vi "Dashboard Main.vi"() -> ()   [LabVIEW 2015]
uses:
  <vilib>/Utility/miscctls.llb/LVRowAndColumnTypeDef.ctl
  <vilib>/event_ctls.llb/eventvkey.ctl
  <vilib>/Rock Robotics/WPI/Dashboard/WPI_DashboardLogging Global.vi
  <vilib>/Utility/config.llb/Write Key (String).vi
  <vilib>/Utility/config.llb/Write Key (I32).vi
  <vilib>/Utility/config.llb/NI_LVConfig.lvlib
panel:
  in  "TCP":refnum<k5>
  in  "Rec Mode":enum32{"Stop", "Record", "Playback"}(radio)
  in  "Vision":u16(ring)=2 items=["Camera Off", "USB Camera SW", "USB Camera HW", "IP Camera"]
  out "Camera IP":string
  out "Image Message":string="Timeout in Camera Communications"
  in  "Dashboard Tab":T1(tab)
  out "Ball in Intake Arm":bool
  in  "Vertical Line (Pixels)":dbl=179.0
  in  "Horizonal Line (Pixels)":dbl=164.0
  in  "Select Auto":string(combo)
  out "NT Connection":bool
  in  "Camera Settings":T2={"Frame Rate"=30, "Compression"=30, "Size"=1} {"Frame Rate" scale=1.0..30.0; "Size" items=["640x480", "320x240", "160x120"]}
  out "Mode":T3(ring)=enum."Auto Disabled"
  in  "DB Camera Config":bool
  out "fps":dbl format="%#.1g"
  out "Mbps":dbl format="%#.1g"
  out "Mbps LED":bool
  in  "Crosshair Color":u32(colorbox)=782080
  out "net address":u32
  out "Numeric":i32
  in  "DB/String 9":string
  in  "DB/String 8":string
  in  "DB/String 7":string
  in  "DB/String 6":string
  in  "DB/String 5":string
  in  "DB/String 4":string
  in  "DB/String 3":string
  in  "DB/String 2":string
  in  "DB/String 1":string
  in  "DB/String 0":string
  in  "DB/Slider 0":dbl(slide) scale=0.0..5.0
  in  "DB/Slider 1":dbl(slide) scale=0.0..5.0
  in  "DB/Slider 2":dbl(slide) scale=0.0..5.0
  in  "DB/Slider 3":dbl(slide) scale=0.0..5.0
  out "DB/LED 3":bool
  out "DB/LED 2":bool
  out "DB/LED 1":bool
  out "DB/LED 0":bool
  in  "DB/Button 3":bool
  in  "DB/Button 2":bool
  in  "DB/Button 1":bool
  in  "DB/Button 0":bool caption="New Name"
  in  "Test Slider":dbl(slide) scale=0.0..100.0 scale format="%#_3g"
  in  "On/Off":bool caption="Solenoid"
  in  "Test Name":u16(ring) items=["Select the test to run..."]
  in  "Test Tree":string(tree)
  in  "Motor":cluster{"Value":dbl, "Enable":bool} {"Value" scale=-1.0..1.0 scale format="%#_3g"}
  out "Progress":T4 {"Test Progress" scale=0.0..100.0}
  in  "Rev/Fwd":cluster{"Forward":bool, "Reverse":bool}
  in  "Test Ring":u16(ring) items=["Monochrome", "Color"]
  out "Cmd Status":string
  in  "Execute Command":bool
  in  "Command Params":string[][](table)
  in  "Command Selection":i32(listbox)
  in  "CheckList":i32(listbox)
  out "Tree":string(tree)
  out "Camera Image":T5(plugin-control)
  out "Background":bool
  # "This tab is a great place for autonomous settings and robot-specific values.\nPlace controls and indicators inside this tab and match name to\nDashboard Variables on robot. You can also delete this comment."
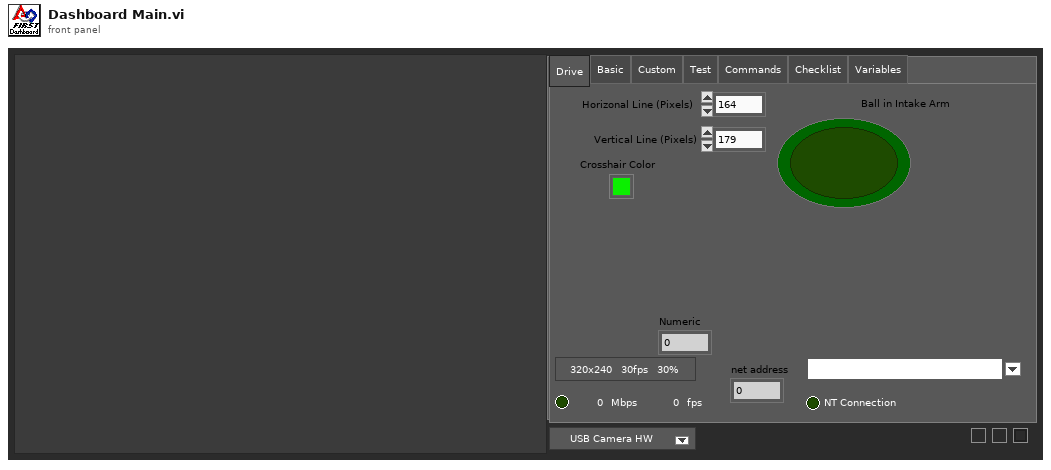
[diagram p1: front panel]
types:
  T1 = enum32{"Drive", "Basic", "Custom", "Test", "Commands", "Checklist", "Variables"}
  T2 = cluster{"Frame Rate":i32, "Compression":i32, "Size":u16}
  T3 = enum8{"Tele-Op Disabled", "Tele-Op Enabled", "Auto Disabled", "Auto Enabled", "Test Disabled", "Test Enabled", "Disconnected", "No Code", "E-Stop"}
  T4 = cluster{"Test Progress":u8, "Test Progress Text":string}
  T5 = typedef "IMAQ Image.ctl" = refnum<image>
  T6 = cluster{"IDs":cluster{"RPC field ID":u16, "Unique ID":u16}, "String":string}
  T7 = enum32{"Drive", "Basic", "Custom", "Test", "Checklist", "Variables"}
  T8 = typedef "Image Type" = u32
  T9 = cluster{"Camera Image":refnum<vi>, "Dashboard Tab":refnum<vi>, "Background":refnum<vi>, "Vision":refnum<vi>, "Rec Mode":refnum<vi>, "Test Slider":refnum<vi>, "On/Off ":refnum<vi>, "Test Ring":refnum<vi>, "Rev/Fwd":refnum<vi>, "Test Name":refnum<vi>, "Motor":refnum<vi>, "Progress":refnum<vi>, "CheckList":refnum<vi>, "Tree":refnum<vi>, "Test Tree":refnum<vi>, "Command Params":refnum<vi>, "Command Selection":refnum<vi>, "Execute Command":refnum<vi>, "Cmd Status":refnum<vi>}
  T10 = cluster{"Error Strings":string, "Disable Counts":cluster{u16, u16}, "Rail Faults":cluster{u16, u16, u16}, "Robot IP":string, "DB Mode":u8, "Event Info":cluster{"Name":string, "Type":u8, "Number":u16, "Replay":u8}, "Camera Addr":string}
  T11 = cluster{"Storage":cluster{"Disk Free":u64, "RAM Block":u32, "RAM free":u32}, "CPU Utilization":cluster{"CPU % ISR":sgl, "CPU % Time Crit":sgl, "CPU % Timed Str":sgl, "CPU % High":sgl, "CPU % Above":sgl, "CPU % Normal":sgl, "CPU % Low":sgl}, "CAN":cluster{"% Bus Utilization":sgl, "Bus Off Cnt":u32, "TX_FIFO Full Cnt":u32, "Receive Error Cnt":u8, "Transmit Error Cnt":u8}, "HID":cluster{"HID Outputs":u32, "Rumble Low":u16, "Rumble High":u16}[]}
  T12 = cluster{"Status bits":cluster{"Test Mode":bool, "Autonomous":bool, "Enabled":bool, "Code Start":bool, "Brownout":bool, "Reserved 2":bool, "Reserved 3":bool, "E-Stop":bool}, "Code Trace":cluster{"Disabled":bool, "TeleOp":bool, "Auto":bool, "Test":bool}, "Controller Type":enum16{"unknown", "cRIO", "roboRio"}, "Code?":enum16{"unknown", "noCode", "code"}, "Battery V":dbl}
  T13 = cluster{"Control Bits":cluster{"TestMode":bool, "Autonomous":bool, "Enabled":bool, "FMS Present":bool, bool, bool, bool, "E-Stop":bool}, "Team Station ":u8, "Countdown":sgl, "Joystick Values":cluster{"Axes":dbl[], "Buttons":bool[], "POVs":i16[]}[]}
  T14 = cluster{"Horizonal Line (Pixels)":dbl, "Horizonal Line (Pixels)":dbl}
  T15 = cluster{"Horizonal Line (Pixels)":dbl, "Vertical Line (Pixels)":dbl}
  T16 = typedef "NI_LVConfig.lvlib/Config Data RefNum.ctl" = refnum<k1>
  T17 = cluster{"Operation":enum16{"Update", "Clear"}, "Color Box":u32}[]
  T18 = typedef "eventvkey.ctl" = enum16{"ASCII", "Enter", "Return", "Shift", "Ctrl", "Alt", "Cmd", "Opt", "Caps", "NumLock", "Clear", "Break", "Up", "Down", "Left", "Right", "Insert", "Delete", "Home", "End", "PageUp", "PageDown", "Escape", "Help", "Pause", "ScrollLock", "F1", "F2", "F3", "F4", "F5", "F6", "F7", "F8", "F9", "F10", "F11", "F12", "F13", "F14", "F15", "F16", "F17", "F18", "F19", "F20", "F21", "F22", "F23", "F24", "Play", "VolumeUp", "VolumeDown", "Mute", "Two Byte Char"}
  T19 = cluster{"Image Size":bool, "Image Type":bool, "Pixel Value":bool, "ROI Information":bool, "Zoom Factor":bool}
  T20 = enum8{"Enabled", "Disabled", "Disabled and Grayed Out"}
  T21 = cluster{"Operation":enum16{"Update", "Clear"}, "Color Box":u32}
  T22 = typedef "LVRowAndColumnTypeDef.ctl" = cluster{"Row":i32, "Column":i32}
  T23 = cluster{"Shift":bool, "Ctrl":bool, "Alt":bool, "Cmd":bool, "Opt":bool}
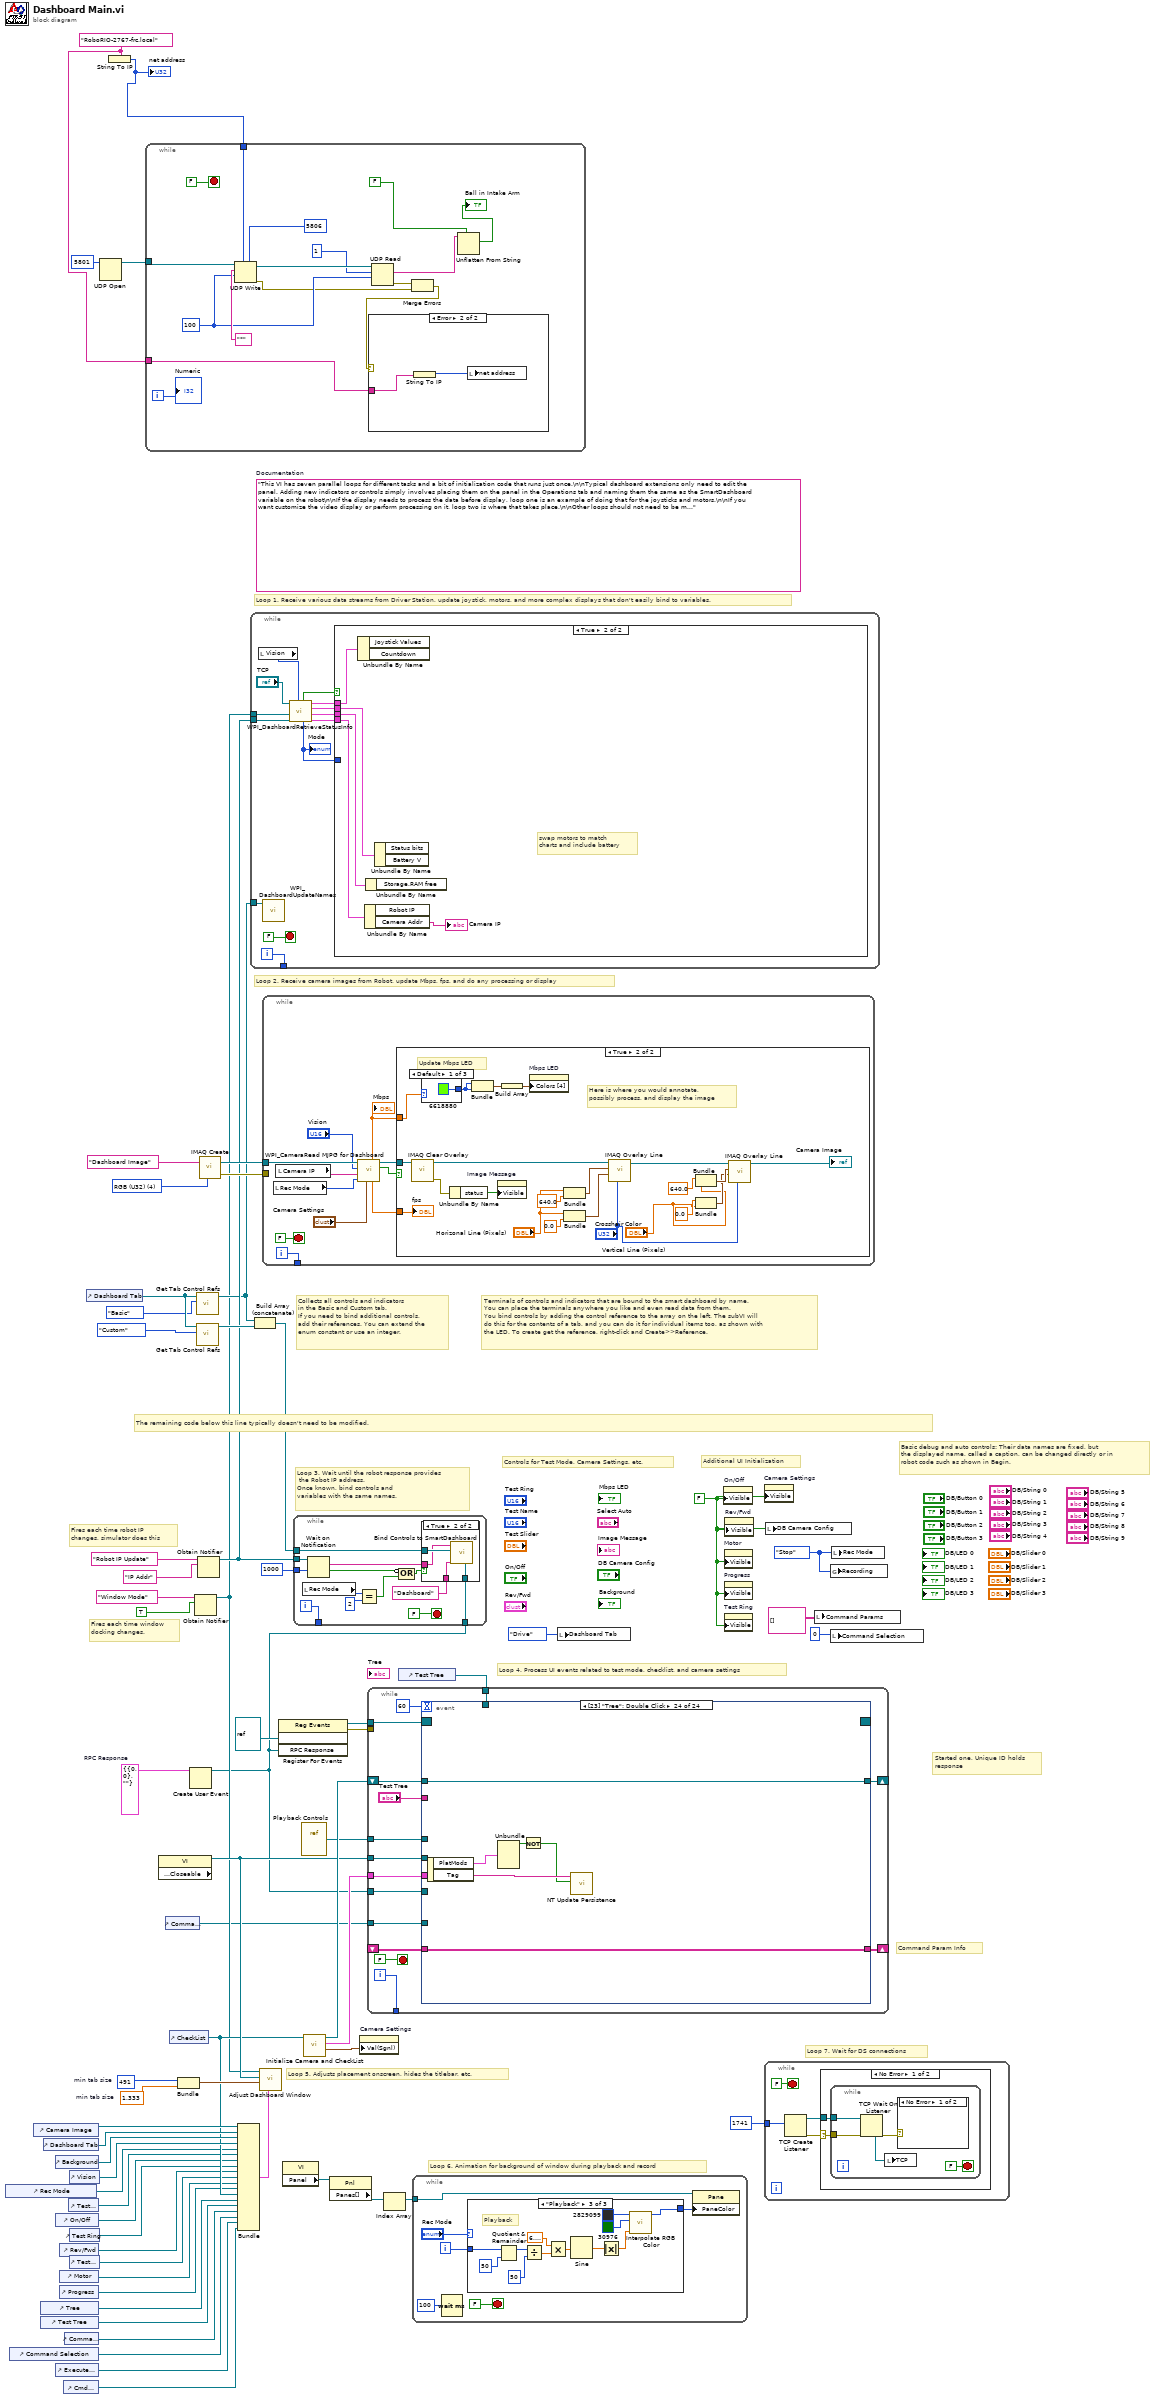
[diagram p0: block diagram]
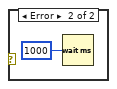
[diagram p3: hidden frame]
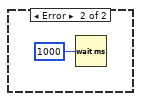
[diagram p4: hidden frame]
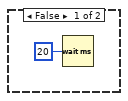
[diagram p5: hidden frame]
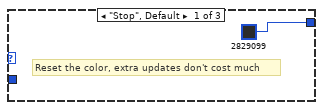
[diagram p6: hidden frame]
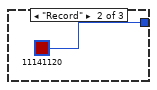
[diagram p7: hidden frame]
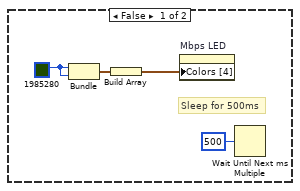
[diagram p9: hidden frame]
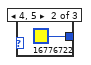
[diagram p10: hidden frame]
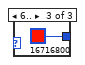
[diagram p11: hidden frame]
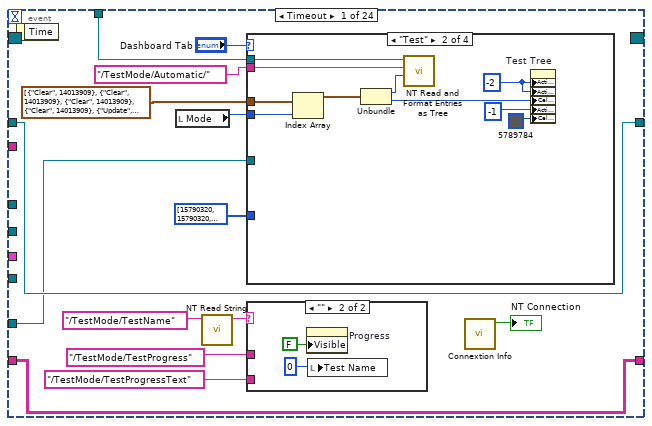
[diagram p12: hidden frame]
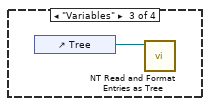
[diagram p14: hidden frame]
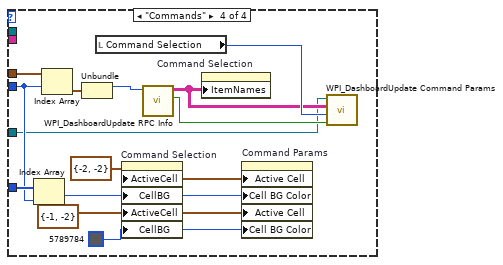
[diagram p15: hidden frame]
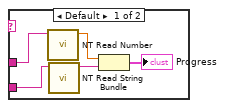
[diagram p16: hidden frame]
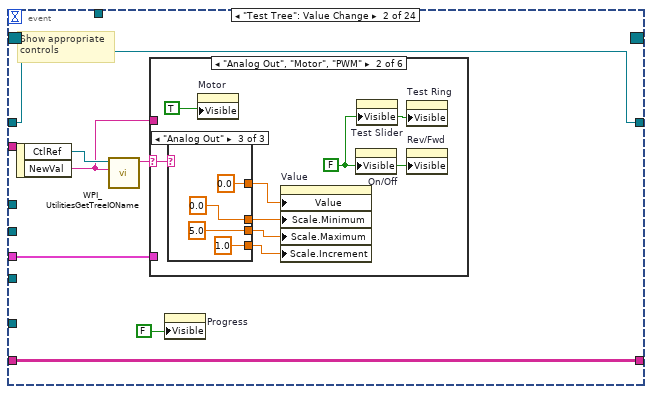
[diagram p17: hidden frame]
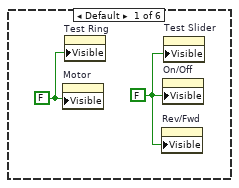
[diagram p18: hidden frame]
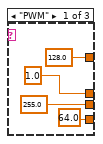
[diagram p19: hidden frame]
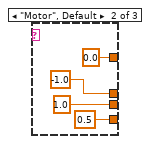
[diagram p20: hidden frame]
diagram:
  w1 = "RoboRIO-2767-frc.local" ("name")
  w11 = T6 {"IDs"={"RPC field ID"=0, "Unique ID"=0}, "String"=""}  # RPC Response
  w37 = 491  # min tab size
  w36 = 1.333  # min tab size
  w45 = enum32{"Stop", "Record", "Playback"}."Stop" ("Rec Mode")
  w19 = FALSE ("Visible")
  (unwired) "This VI has seven parallel loops for different tasks and a bit of initialization code that runs just once.\n\nTypical dashboard extensions only need to edit the panel. Adding new indicators or controls simply involves placing them on the panel in the Operations tab and naming them the same as the SmartDashboard variable on the robot\n\nIf the display needs to process the data before display, loop one is an example of doing that for the joysticks and motors.\n\nIf you want customize the video display or perform processing on it, loop two is where that takes place.\n\nOther loops should not need to be modified. They are pretty standard, and document the task they perform."  # Documentation
  w65 = T8 4 items=["Grayscale (U8)", "Grayscale (I16)", "Grayscale (SGL)", "Complex (CSG)", "RGB (U32)", "HSL (U32)", "RGB (U64)"] ("Image Type")
  # "Command Param Info"
  # "Started one, Unique ID holds\nresponse"
  # "Loop 7. Wait for DS connections"
  # "Basic debug and auto controls: Their data names are fixed, but\nthe displayed name, called a caption, can be changed directly or in\nrobot code such as shown in Begin."
  # "Controls for Test Mode, Camera Settings, etc."
  # "Additional UI Initialization"
  # "Loop 6. Animation for background of window during playback and record"
  # "Fires each time robot IP\nchanges, simulator does this"
  # "Fires each time window\ndocking changes."
  # "Collects all controls and indicators\nin the Basic and Custom tab.\nIf you need to bind additional controls,\nadd their references. You can extend the\nenum constant or use an integer."
  # "The remaining code below this line typically doesn't need to be modified."
  # "Loop 4. Process UI events related to test mode, checklist, and camera settings"
  # "Terminals of controls and indicators that are bound to the smart dashboard by name.\nYou can place the terminals anywhere you like and even read data from them.\nYou bind controls by adding the control reference to the array on the left. The subVI will\ndo this for the contents of a tab, and you can do it for individual items too, as shown with\nthe LED. To create get the reference, right-click and Create>>Reference."
  # "Loop 3. Wait until the robot response provides\n the Robot IP address.\nOnce known, bind controls and\nvariables with the same names."
  # "Loop 5. Adjusts placement onscreen, hides the titlebar, etc."
  # "Loop 1. Receive various data streams from Driver Station, update joystick, motors, and more complex displays that don't easily bind to variables."
  # "Loop 2. Receive camera images from Robot, update Mbps, fps, and do any processing or display"
  n1 = control-ref of="Rec Mode"() -> (w25:refnum<vi>)
  n2 = control-ref of="Command Selection"() -> (w10:refnum<vi>)
  n3 = control-ref of="Camera Image"() -> (w40:refnum<vi>)
  n4 = control-ref of="Tree"() -> (w29:refnum<vi>)
  n5 = control-ref of="Test Tree"() -> (w28:refnum<vi>)
  n6 = control-ref of="Dashboard Tab"() -> (w39:refnum<vi>)
  n7 = control-ref of="Execute Command"() -> (w12:refnum<vi>)
  n8 = control-ref of="Background"() -> (w34:refnum<vi>)
  n9 = control-ref of="On/Off"() -> (w23:refnum<vi>)
  n10 = control-ref of="Progress"() -> (w20:refnum<vi>)
  n11 = control-ref of="Rev/Fwd"() -> (w21:refnum<vi>)
  n12 = control-ref of="Motor"() -> (w26:refnum<vi>)
  n13 = control-ref of="Cmd Status"() -> (w6:refnum<vi>)
  n14 = control-ref of="Command Params"() -> (w13:refnum<vi>)
  n15 = control-ref of="Test Slider"() -> (w24:refnum<vi>)
  n16 = control-ref of="Vision"() -> (w38:refnum<vi>)
  n17 = control-ref of="Test Ring"() -> (w22:refnum<vi>)
  n18 = control-ref of="Test Name"() -> (w27:refnum<vi>)
  n19 = control-ref of="Dashboard Tab"() -> (w43:refnum<vi>)
  n20 = UDP Open(11:u16 5801 ("port")) -> (port=w3:refnum<k16>)  [unwired: 4 in, 2 out]
  n21 = String To IP(1:w1) -> (0:w2:u32)
  "net address" <- w2
  n22 = while {
    tunnel: w3 -> [w79]
    tunnel: w2 -> [w70]
    tunnel: w1 -> [w66]
    i -> [w72]
    stop <- FALSE stop-if-true
    w71 = 100 ("timeout ms (25000)")
    n23 = UDP Write(address=w70, port or service name=u16 5806, connection ID=w79, data in="*", 9:w71) -> (error out=w68:errorcluster, 3:w77:refnum<k16>)  [unwired: 1 in]
    n24 = UDP Read(connection ID=w77, max size (548)=1, timeout ms (25000)=w71) -> (data out=w74:string, error out=w69:errorcluster)  [unwired: 1 in, 3 out]
    n25 = Merge Errors(w69, w68) -> (w67:errorcluster)
    n26 = case shown="Error" w67 {
      tunnel: w66 -> [_ w82]
      frame No Error {
      }
      frame Error {
        n27 = String To IP(1:w82) -> (0:w83:u32)
        n28 = local write "net address"(w83) -> ()
      }
    }
    n29 = Unflatten From String(type=FALSE ("Boolean"), binary string=w74) -> (value=→"Ball in Intake Arm":bool)  [unwired: 3 in, 2 out]
    "Numeric" <- w72
  }
  n30 = property class="VI" props=["Front Panel.Closeable"]() -> (reference out=w44:refnum<vi>)  [unwired: 2 in, 2 out]
  n31 = control-ref of="Command Params"() -> (w5:refnum<vi>)
  n32 = control-ref of="CheckList"() -> (w30:refnum<vi>)
  n33 = Bundle("min tab size"=w37, "min tab size"=w36) -> (w35:cluster{"min tab size":i32, "min tab size":dbl})  [unwired: 1 in]
  n34 = Create User Event(user event datatype=w11) -> (user event=w7:refnum<user-event>)  [unwired: 1 in, 1 out]
  n35 = Obtain Notifier(name (unnamed)="Window Mode", notification data type=TRUE) -> (notifier out=w16:refnum<notifier>)  [unwired: 2 in, 2 out]
  n36 = call <vilib>:"Get Tab Control Refs.vi"("Page Index"=T7."Basic" ("Dashboard Tab"), "TabControl in"=w43) -> ("ControlsOnPage"=w17:refnum<vi>[])  [unwired: 9 in]
  n37 = call <vilib>:"Get Tab Control Refs.vi"("Page Index"=T7."Custom" ("Dashboard Tab"), "TabControl in"=w43) -> ("ControlsOnPage"=w42:refnum<vi>[])  [unwired: 9 in]
  n38 = Obtain Notifier(name (unnamed)="Robot IP Update", notification data type="IP Addr" ("name (unnamed)")) -> (notifier out=w18:refnum<notifier>)  [unwired: 2 in, 2 out]
  n39 = call "IMAQ Create"("Image Name"="Dashboard Image", "Image Type"=w65) -> ("New Image"=w63:T5, "error out"=w62:errorcluster)  [unwired: 2 in, 1 out]
  n40 = Bundle("Camera Image"=w40, "Dashboard Tab"=w39, "Background"=w34, "Vision"=w38, "Rec Mode"=w25, "Test Slider"=w24, "On/Off"=w23, "Test Ring"=w22, "Rev/Fwd"=w21, "Test Name"=w27, "Motor"=w26, "Progress"=w20, "CheckList"=w30, "Tree"=w29, "Test Tree"=w28, "Command Params"=w13, "Command Selection"=w10, "Execute Command"=w12, "Cmd Status"=w6) -> (w31:T9)  [unwired: 1 in]
  n41 = while {
    tunnel: [w95] -> _
    tunnel: w18 -> [w89]
    tunnel: w17 -> [w88]
    tunnel: w16 -> [w84]
    i -> [w95]
    stop <- FALSE stop-if-true
    n42 = local read "Vision"() -> (w86:u16)
    n43 = call <vilib>:"WPI_DashboardUpdateNames.vi"("Controls on Tab"=w88) -> ()  [unwired: 11 in]
    n44 = call <vilib>:"WPI_DashboardRetrieveStatusInfo.vi"("Vision"=w86, "Binding Refnum"=w89, "Window Mode Notifier"=w84, "TCP Cnx"="TCP") -> ("Power and Errors"=w90:T10, "Robot Metrics"=w93:T11, "Status Info"=w94:T12, "Control Info"=w91:T13, "Robot Mode"=w87:T3, "Process?"=w92:bool)  [unwired: 2 in]
    "Mode" <- w87
    n45 = case shown="True" w92 {
      tunnel: w94 -> [_ w102]
      tunnel: w93 -> [_ w101]
      tunnel: w91 -> [_ w100]
      tunnel: w90 -> [_ w99]
      tunnel: w87 -> [_ _]
      frame False {
        n46 = Wait (ms)(milliseconds to wait=u32 20) -> ()  [unwired: 1 out]
      }
      frame True {
        # "swap motors to match\ncharts and include battery"
        n47 = Unbundle By Name(w100) -> ()  [unwired: 2 out]
        n48 = Unbundle By Name(w99) -> ("Camera Addr"=→"Camera IP":string)  [unwired: 1 out]
        n49 = Unbundle By Name(w101) -> ()  [unwired: 1 out]
        n50 = Unbundle By Name(w102) -> ()  [unwired: 2 out]
      }
    }
  }
  n51 = Build Array (concatenate)(w17, w42) -> (w41:refnum<vi>[])
  n52 = call "Adjust Dashboard Window.vi"("Sizing Refnums"=w31, "Size Constraints"=w35, "VI"=w44, "WIn Mode"=w16) -> ()  [unwired: 8 in]
  n53 = while {
    tunnel: w63 -> [w111]
    tunnel: w62 -> [_]
    tunnel: [w112] -> _
    i -> [w112]
    stop <- FALSE stop-if-true
    n54 = local read "Rec Mode"() -> (w106:enum32{"Stop", "Record", "Playback"})
    n55 = local read "Camera IP"() -> (w104:string)
    n56 = call <vilib>:"WPI_CameraRead MJPG for Dashboard.vi"("Camera Settings"="Camera Settings", "Rec Mode"=w106, "Camera IP"=w104, "Camera Mode"="Vision", "Refnum in"=w111) -> ("Active"=w109:bool, "Refnum out"=w110:T5, "FPS"=w108:dbl, "Bandwidth (Mbps)"=w103:dbl)  [unwired: 3 in]
    "Mbps" <- w103
    n57 = case shown="True" w109 {
      tunnel: w110 -> [_ w134]
      tunnel: w103 -> [_ w133]
      tunnel: w108 -> [_ w132]
      frame False {
        w114 = u32 1985280 ("Color Box")
        # "Sleep for 500ms"
        n58 = Bundle("Color Box"=w114, "Color Box"=w114) -> (w116:cluster{"Color Box":u32, "Color Box":u32})  [unwired: 1 out]
        n59 = Build Array(w116) -> (w115:cluster{"Color Box":u32, "Color Box":u32}[])
        n60 = property on="Mbps LED" class="Bool (strict)"("Colors [4]"=w115) -> ()  [unwired: 2 in, 2 out]
        n61 = Wait Until Next ms Multiple(millisecond multiple=u32 500) -> ()  [unwired: 1 out]
      }
      frame True {
        # "Here is where you would annotate,\npossibly process, and display the image"
        # "Update Mbps LED"
        n62 = call "IMAQ Clear Overlay"("Image"=w134) -> ("error out"=w138:errorcluster, "Image Out"=w131:T5)  [unwired: 2 in, 7 out]
        n63 = case shown="Default" w133 {
          tunnel: [u32 6618880 ("Color Box") u32 16776722 ("Color Box") u32 16716800 ("Color Box")] -> w135
          frame Default {
          }
          frame 4, 5 {
          }
          frame 6.. {
          }
        }
        n64 = Unbundle By Name(w138) -> ("status"=w139:bool)
        n65 = Bundle("Color Box"=w135, "Color Box"=w135) -> (w137:cluster{"Color Box":u32, "Color Box":u32})  [unwired: 1 out]
        n66 = property on="Image Message" class="Str"("Visible"=w139) -> ()  [unwired: 2 in, 2 out]
        n67 = Build Array(w137) -> (w136:cluster{"Color Box":u32, "Color Box":u32}[])
        n68 = property on="Mbps LED" class="Bool (strict)"("Colors [4]"=w136) -> ()  [unwired: 2 in, 2 out]
        n69 = Bundle("Horizonal Line (Pixels)"="Horizonal Line (Pixels)", "Horizonal Line (Pixels)"=640.0) -> (w127:T14)  [unwired: 1 in]
        n70 = Bundle("Horizonal Line (Pixels)"="Horizonal Line (Pixels)", "Horizonal Line (Pixels)"=0.0) -> (w126:T14)  [unwired: 1 in]
        n71 = call "IMAQ Overlay Line"("Color"="Crosshair Color", "End Point"=w126, "Start Point"=w127, "Image"=w131) -> ("Image Out"=w119:T5)  [unwired: 6 in, 1 out]
        n72 = Bundle("Horizonal Line (Pixels)"=640.0, "Vertical Line (Pixels)"="Vertical Line (Pixels)") -> (w125:T15)  [unwired: 1 in]
        n73 = Bundle("Horizonal Line (Pixels)"=0.0, "Vertical Line (Pixels)"="Vertical Line (Pixels)") -> (w124:T15)  [unwired: 1 in]
        n74 = call "IMAQ Overlay Line"("Color"="Crosshair Color", "End Point"=w124, "Start Point"=w125, "Image"=w119) -> ("Image Out"=→"Camera Image":T5)  [unwired: 6 in, 1 out]
        "fps" <- w132
      }
    }
  }
  n75 = register-events(refnum<vi> refnum, w7) -> (reference out=w49:refnum<event-registration>, error out=w48:errorcluster)  [unwired: 2 in]
  n76 = property class="VI"() -> ("Panel"=w52:refnum<vi>)  [unwired: 2 in, 2 out]
  n77 = while {
    tunnel: w41 -> [w155]
    tunnel: w18 -> [w153]
    tunnel: [w151] -> _
    tunnel: u32 1000 ("milliseconds to wait") -> [w150]
    tunnel: w7 -> [w143]
    i -> [w151]
    stop <- FALSE stop-if-true
    n78 = local read "Rec Mode"() -> (w146:enum32{"Stop", "Record", "Playback"})
    n79 = Wait on Notification(notifier=w153, timeout in ms (-1)=w150) -> (notification=w152:string, timed out?=w148:bool)  [unwired: 2 in, 2 out]
    n80 = Equal?(x=w146, y=u16 2 ("Rec Mode")) -> (x = y?=w147:bool)
    n81 = Compound Arithmetic op=OR(invert w148, w147) -> (w149:bool)
    n82 = case shown="True" w149 {
      tunnel: w155 -> [_ w159]
      tunnel: w152 -> [_ w158]
      tunnel: "Dashboard" -> [_ w157]
      tunnel: w143 -> [_ w156]
      frame False {
      }
      frame True {
        n83 = call <vilib>:"Bind Controls to SmartDashboard.vi"("RPC ref"=w156, "Client Name"=w157, "Bound Control Refs"=w159, "Server IP Address"=w158) -> ()  [unwired: 8 in]
      }
    }
  }
  n84 = vi-ref "Playback Controls.vi"() -> (w50:refnum<vi>)
  n85 = call "Initialize Camera and CheckList.vi"("ListBox in"=w30) -> ("Cluster"=w56:cluster{"value":i32, "value":i32, "index":i32}, "Array"=w57:cluster{string[]}[], "File Refnum"=w55:T16)  [unwired: 8 in]
  n86 = property class="Pnl"(reference=w52) -> ("Panes[]"=w53:refnum<vi>[])  [unwired: 1 in, 2 out]
  n87 = property on="Camera Settings" class="Clust (strict)"("Val(Sgnl)"=w56) -> ()  [unwired: 2 in, 2 out]
  n88 = Index Array(array=w53) -> (element=w51:refnum<vi>)  [unwired: 1 in]
  n89 = control-ref of="Test Tree"() -> (w54:refnum<vi>)
  n90 = while {
    tunnel: w57 -> [w171]
    shift-right: [w170] -> _
    shift-left: w55 -> [w169]
    tunnel: [w168] -> _
    tunnel: w54 -> [w167]
    tunnel: w50 -> [w166]
    tunnel: w49 -> [w165]
    tunnel: w48 -> [_]
    tunnel: w44 -> [w164]
    tunnel: w7 -> [w163]
    tunnel: w5 -> [w162]
    shift-right: [w161] -> _
    shift-left: _ -> [w160]
    i -> [w168]
    stop <- FALSE stop-if-true
    n91 = event shown="[23] \"Tree\": Double Click" {
      selector: w165 -> [_ _ _ _ _ _ _ _ _ _ _ _ _ _ _ _ _ _ _ _ _ _ _ _]
      dyn-events: [_ _ _ _ _ _ _ _ _ _ _ _ _ _ _ _ _ _ w480 _ _ _ _ _] -> _
      timeout: u32 60 ("milliseconds to wait") -> [_ _ _ _ _ _ _ _ _ _ _ _ _ _ _ _ _ _ _ _ _ _ _ _]
      tunnel: w167 -> [w184 _ _ _ _ _ _ _ _ _ _ _ _ _ _ _ _ _ _ _ _ _ _ _]
      tunnel: "Test Tree" -> [_ _ _ _ _ _ _ _ _ _ _ _ _ w443 w452 w455 w460 w469 _ _ _ _ _ _]
      tunnel: w171 -> [_ w222 _ _ _ _ _ _ _ _ _ w405 w436 _ _ _ _ _ _ _ _ _ _ _]
      tunnel: [w181 w221 w325 w331 w341 w345 w351 w363 w371 w377 w390 w404 w429 w442 w450 w454 w459 w468 w482 w498 w500 w508 w519 w524] -> w170
      tunnel: w169 -> [w181 w221 w325 w331 w341 w345 w351 w363 w371 w377 w390 w403 w429 w442 w450 w454 w459 w468 w482 w498 w500 w508 w519 w524]
      tunnel: w166 -> [_ _ _ _ _ _ _ _ _ _ _ _ _ _ _ _ _ _ w483 _ w503 _ _ _]
      tunnel: w164 -> [_ _ _ _ _ _ _ _ _ _ _ _ _ _ _ _ _ _ w478 _ _ _ _ _]
      tunnel: w163 -> [_ _ _ _ _ _ _ _ _ _ _ _ _ _ _ _ _ _ w474 _ _ _ _ _]
      tunnel: w162 -> [w176 _ _ _ _ _ w349 _ _ _ _ _ _ _ _ _ _ _ _ _ _ _ _ _]
      tunnel: [w175 w220 w324 w330 w340 w346 w347 w357 w368 w376 w389 w402 w428 w441 w449 w453 w458 w467 w473 w496 w499 w504 w512 w525] -> w161
      tunnel: w160 -> [w175 w220 w324 w330 w340 w346 w347 _ _ w376 w389 w402 w428 w441 w449 w453 w458 w467 w473 w496 w499 w504 w512 w525]
      event Timeout {
        n92 = event-data() -> ()  [unwired: 1 in, 1 out]
        n93 = local read "Mode"() -> (w178:T3)
        n94 = call <vilib>:"NT Read String.vi"("Name"="/TestMode/TestName") -> ("String"=w187:string)  [unwired: 9 in, 1 out]
        n95 = case shown="\"Test\"" "Dashboard Tab" {
          tunnel: w184 -> [_ w198 _ _]
          tunnel: "/TestMode/Automatic/" ("Name Pattern") -> [_ w197 _ _]
          tunnel: T17 [{"Operation"=enum."Clear", "Color Box"=14013909}, {"Operation"=enum."Clear", "Color Box"=14013909}, {"Operation"=enum."Clear", "Color Box"=14013909}, {"Operation"=enum."Clear", "Color Box"=14013909}, {"Operation"=enum."Update", "Color Box"=14013909}, {"Operation"=enum."Update", "Color Box"=16777215}, {"Operation"=enum."Clear", "Color Box"=14013909}, {"Operation"=enum."Clear", "Color Box"=14013909}, {"Operation"=enum."Clear", "Color Box"=14013909}] -> [_ w190 _ w207]
          tunnel: w178 -> [_ w189 _ w206]
          tunnel: u32[] [15790320, 15790320, 15790320, 15790320, 16777215, 16777215, 15790320, 15790320, 15790320] -> [_ _ _ w212]
          tunnel: w176 -> [_ _ _ w200]
          frame "Custom", Default {
          }
          frame "Test" {
            w196 = -2 ("Active Item:Row Number")
            n96 = Index Array(array=w190, index=w189) -> (element=w191:T21)
            n97 = Unbundle(w191) -> ("Operation"=w192:enum16{"Update", "Clear"}, "Color Box"=w193:u32)
            n98 = call <vilib>:"NT Read and Format Entries as Tree.vi"("Operation"=w192, "Name Pattern"=w197, "Tree Refnum"=w198) -> ()  [unwired: 7 in, 2 out]
            n99 = property on="Test Tree" class="Tree (strict)"("Active Item Row Number"=w196, "ActiveColNum"=w196, "CellBG"=w193, "Active Item Row Number"=-1 ("Active Item:Row Number"), "CellBG"=u32 5789784 ("Color Box")) -> ()  [unwired: 2 in, 2 out]
          }
          frame "Variables" {
            n100 = control-ref of="Tree"() -> (w199:refnum<vi>)
            n101 = call <vilib>:"NT Read and Format Entries as Tree.vi"("Tree Refnum"=w199) -> ()  [unwired: 9 in, 2 out]
          }
          frame "Commands" {
            w208 = u32 5789784 ("Color Box")
            w209 = T22 {"Row"=-1, "Column"=-2} ("Active Cell:Active Cell")
            w211 = T22 {"Row"=-2, "Column"=-2} ("Active Cell:Active Cell")
            n102 = Index Array(array=w212, index=w206) -> (element=w210:u32)
            n103 = Index Array(array=w207, index=w206) -> (element=w205:T21)
            n104 = Unbundle(w205) -> ("Operation"=w204:enum16{"Update", "Clear"})  [unwired: 1 out]
            n105 = local read "Command Selection"() -> (w203:i32)
            n106 = property on="Command Selection" class="MCListbox (strict)"("ActiveCell"=w211, "CellBG"=w210, "ActiveCell"=w209, "CellBG"=w208) -> ()  [unwired: 2 in, 2 out]
            n107 = call <vilib>:"WPI_DashboardUpdate RPC Info.vi"("Operation"=w204) -> ("update"=w202:bool, "commands"=w201:string[][])  [unwired: 9 in]
            n108 = property on="Command Selection" class="MCListbox (strict)"("ItemNames"=w201) -> ()  [unwired: 2 in, 2 out]
            n109 = property on="Command Params" class="Tbl (strict)"("Active Cell"=w211, "Cell BG Color"=w210, "Active Cell"=w209, "Cell BG Color"=w208) -> ()  [unwired: 2 in, 2 out]
            n110 = call <vilib>:"WPI_DashboardUpdate Command Params.vi"("Update"=w202, "NewVal"=w203, "Commands"=w201, "Param Tbl"=w200) -> ()  [unwired: 7 in, 1 out]
          }
        }
        n111 = case shown="\"\"" w187 {
          tunnel: "/TestMode/TestProgress" ("Name") -> [w214 _]
          tunnel: "/TestMode/TestProgressText" ("Name") -> [w213 _]
          frame Default {
            n112 = call <vilib>:"NT Read Number.vi"("Name"=w214) -> ("Numeric"=w215:dbl)  [unwired: 9 in, 1 out]
            n113 = call <vilib>:"NT Read String.vi"("Name"=w213) -> ("String"=w216:string)  [unwired: 9 in, 1 out]
            n114 = Bundle("Numeric"=w215, "String"=w216) -> (→"Progress":cluster{"Numeric":dbl, "String":string})  [unwired: 1 in]
          }
          frame "" {
            n115 = property on="Progress" class="Clust (strict)"("Visible"=FALSE) -> ()  [unwired: 2 in, 2 out]
            n116 = local write "Test Name"(u16 0) -> ()
          }
        }
        n117 = call <vilib>:"Connextion Info.vi"() -> ("Connected"=→"NT Connection":bool)  [unwired: 10 in, 1 out]
      }
      event "Test Tree": Value Change {
        # "Show appropriate\ncontrols"
        n118 = event-data() -> ("CtlRef"=w225:refnum<vi>, "NewVal"=w223:string)  [unwired: 1 in]
        n119 = call <vilib>:"WPI_UtilitiesGetTreeIOName.vi"("NewVal"=w223, "TreeControl in"=w225) -> ("I/O Name"=w226:string)  [unwired: 9 in]
        n120 = case shown="\"Analog Out\", \"Motor\", \"PWM\"" w226 {
          selector: w226 -> [_ w233 _ w255 w264 _]
          tunnel: w223 -> [_ _ w252 w254 _ w271]
          tunnel: w222 -> [_ _ _ _ _ w270]
          frame Default {
            w228 = FALSE ("Visible")
            w227 = FALSE ("Visible")
            n121 = property on="Motor" class="Clust (strict)"("Visible"=w227) -> ()  [unwired: 2 in, 2 out]
            n122 = property on="Test Ring" class="Ring (strict)"("Visible"=w227) -> ()  [unwired: 2 in, 2 out]
            n123 = property on="Rev/Fwd" class="Clust (strict)"("Visible"=w228) -> ()  [unwired: 2 in, 2 out]
            n124 = property on="On/Off" class="Bool (strict)"("Visible"=w228) -> ()  [unwired: 2 in, 2 out]
            n125 = property on="Test Slider" class="Slide (strict)"("Visible"=w228) -> ()  [unwired: 2 in, 2 out]
          }
          frame "Analog Out", "Motor", "PWM" {
            w234 = FALSE ("Visible")
            n126 = case shown="\"Analog Out\"" w233 {
              tunnel: [1.0 ("Value") -1.0 ("Value") 0.0 ("Value")] -> w232
              tunnel: [255.0 ("Value") 1.0 ("Value") 5.0 ("Value")] -> w231
              tunnel: [128.0 ("Value") 0.0 ("Value") 0.0 ("Value")] -> w230
              tunnel: [64.0 ("Value") 0.5 ("Value") 1.0 ("Value")] -> w229
              frame "PWM" {
              }
              frame "Motor", Default {
              }
              frame "Analog Out" {
              }
            }
            n127 = property on="Motor" class="Clust (strict)"("Visible"=TRUE) -> ()  [unwired: 2 in, 2 out]
            n128 = property on="Value" class="Slide (strict)"("Value"=w230, "Scale.Minimum"=w232, "Scale.Maximum"=w231, "Scale.Increment"=w229) -> ()  [unwired: 2 in, 2 out]
            n129 = property on="On/Off" class="Bool (strict)"("Visible"=w234) -> ()  [unwired: 2 in, 2 out]
            n130 = property on="Test Slider" class="Slide (strict)"("Visible"=w234) -> ()  [unwired: 2 in, 2 out]
            n131 = property on="Test Ring" class="Ring (strict)"("Visible"=w234) -> ()  [unwired: 2 in, 2 out]
            n132 = property on="Rev/Fwd" class="Clust (strict)"("Visible"=w234) -> ()  [unwired: 2 in, 2 out]
          }
          frame "Servo" {
            w250 = FALSE ("Visible")
            n133 = call <vilib>:"NT Read Number.vi"("Name"=w252) -> ("Numeric"=w251:dbl)  [unwired: 9 in, 1 out]
            n134 = property on="Test Slider" class="Slide (strict)"("Visible"=TRUE, "Scale.Maximum"=170.0 ("Scale.Range:Maximum")) -> ()  [unwired: 2 in, 2 out]
            n135 = local write "Test Slider"(w251) -> ()
            n136 = property on="Motor" class="Clust (strict)"("Visible"=w250) -> ()  [unwired: 2 in, 2 out]
            n137 = property on="Rev/Fwd" class="Clust (strict)"("Visible"=w250) -> ()  [unwired: 2 in, 2 out]
            n138 = property on="On/Off" class="Bool (strict)"("Visible"=w250) -> ()  [unwired: 2 in, 2 out]
            n139 = property on="Test Ring" class="Ring (strict)"("Visible"=w250) -> ()  [unwired: 2 in, 2 out]
          }
          frame "Relay", "Solenoid" {
            w253 = FALSE ("Visible")
            n140 = property on="Motor" class="Clust (strict)"("Visible"=w253) -> ()  [unwired: 2 in, 2 out]
            n141 = property on="Test Slider" class="Slide (strict)"("Visible"=w253) -> ()  [unwired: 2 in, 2 out]
            n142 = Search and Replace String(input string=w254, search string="/Value  **", replace string="/Direction") -> (result string=w260:string)  [unwired: 5 in, 3 out]
            n143 = property on="Test Ring" class="Ring (strict)"("Visible"=w253) -> ()  [unwired: 2 in, 2 out]
            n144 = call <vilib>:"NT Read String.vi"("Name"=w260) -> ("String"=w258:string)  [unwired: 9 in, 1 out]
            n145 = Equal?(x="Both directions", y=w258) -> (x = y?=w256:bool)
            n146 = Not(x=w256) -> (.not. x?=w257:bool)
            n147 = property on="Rev/Fwd" class="Clust (strict)"("Visible"=w256) -> ()  [unwired: 2 in, 2 out]
            n148 = property on="On/Off" class="Bool (strict)"("Visible"=w257, "Caption.Text"=w255) -> ()  [unwired: 2 in, 2 out]
          }
          frame "Compressor", "Digital Out" {
            w263 = FALSE ("Visible")
            # "Get direction and finish"
            n149 = property on="Motor" class="Clust (strict)"("Visible"=w263) -> ()  [unwired: 2 in, 2 out]
            n150 = property on="Test Slider" class="Slide (strict)"("Visible"=w263) -> ()  [unwired: 2 in, 2 out]
            n151 = property on="Test Ring" class="Ring (strict)"("Visible"=w263) -> ()  [unwired: 2 in, 2 out]
            n152 = property on="On/Off" class="Bool (strict)"("Visible"=TRUE, "Caption.Text"=w264) -> ()  [unwired: 2 in, 2 out]
            n153 = property on="Rev/Fwd" class="Clust (strict)"("Visible"=FALSE) -> ()  [unwired: 2 in, 2 out]
          }
          frame "Camera" {
            n154 = call <vilib>:"Get Last Path Segment.vi"("String in"=w271) -> ("String out"=w272:string)  [unwired: 10 in]
            n155 = property on="On/Off" class="Bool (strict)"("Visible"=FALSE) -> ()  [unwired: 2 in, 2 out]
            n156 = property on="Motor" class="Clust (strict)"("Visible"=FALSE) -> ()  [unwired: 2 in, 2 out]
            n157 = property on="Rev/Fwd" class="Clust (strict)"("Visible"=FALSE) -> ()  [unwired: 2 in, 2 out]
            n158 = case shown="\"White Balance  **\"" w272 {
              tunnel: w271 -> [w278 w287 w296 w305 w314 _ w320]
              tunnel: w270 -> [w276 w284 w293 w302 w311 _ _]
              frame "Size  **" {
                n159 = Index Array(array=w276) -> (element=w275:cluster{string[]})  [unwired: 1 in]
                n160 = call <vilib>:"NT Read String.vi"("Name"=w278) -> ("String"=w277:string)  [unwired: 9 in, 1 out]
                n161 = Unbundle(w275) -> (w273:string[])
                n162 = Match First String(2:w273, 3:w277) -> (0:w274:i32)  [unwired: 1 out]
                n163 = property on="Test Ring" class="Ring (strict)"("Value"=w274, "Strings []"=w273) -> ()  [unwired: 2 in, 2 out]
                n164 = property on="Test Ring" class="Ring (strict)"("Visible"=TRUE) -> ()  [unwired: 2 in, 2 out]
                n165 = property on="Test Slider" class="Slide (strict)"("Visible"=FALSE) -> ()  [unwired: 2 in, 2 out]
              }
              frame "White Balance  **" {
                n166 = Index Array(array=w284, index=1) -> (element=w285:cluster{string[]})
                n167 = call <vilib>:"NT Read String.vi"("Name"=w287) -> ("String"=w286:string)  [unwired: 9 in, 1 out]
                n168 = Unbundle(w285) -> (w282:string[])
                n169 = Match First String(2:w282, 3:w286) -> (0:w281:i32)  [unwired: 1 out]
                n170 = property on="Test Ring" class="Ring (strict)"("Value"=w281, "Strings []"=w282) -> ()  [unwired: 2 in, 2 out]
                n171 = property on="Test Ring" class="Ring (strict)"("Visible"=TRUE) -> ()  [unwired: 2 in, 2 out]
                n172 = property on="Test Slider" class="Slide (strict)"("Visible"=FALSE) -> ()  [unwired: 2 in, 2 out]
              }
              frame "Exposure  **" {
                n173 = Index Array(array=w293, index=2) -> (element=w294:cluster{string[]})
                n174 = call <vilib>:"NT Read String.vi"("Name"=w296) -> ("String"=w295:string)  [unwired: 9 in, 1 out]
                n175 = Unbundle(w294) -> (w290:string[])
                n176 = Match First String(2:w290, 3:w295) -> (0:w291:i32)  [unwired: 1 out]
                n177 = property on="Test Ring" class="Ring (strict)"("Value"=w291, "Strings []"=w290) -> ()  [unwired: 2 in, 2 out]
                n178 = property on="Test Ring" class="Ring (strict)"("Visible"=TRUE) -> ()  [unwired: 2 in, 2 out]
                n179 = property on="Test Slider" class="Slide (strict)"("Visible"=FALSE) -> ()  [unwired: 2 in, 2 out]
              }
              frame "Exposure Priority  **" {
                n180 = Index Array(array=w302, index=3) -> (element=w303:cluster{string[]})
                n181 = call <vilib>:"NT Read String.vi"("Name"=w305) -> ("String"=w304:string)  [unwired: 9 in, 1 out]
                n182 = Unbundle(w303) -> (w299:string[])
                n183 = Match First String(2:w299, 3:w304) -> (0:w300:i32)  [unwired: 1 out]
                n184 = property on="Test Ring" class="Ring (strict)"("Value"=w300, "Strings []"=w299) -> ()  [unwired: 2 in, 2 out]
                n185 = property on="Test Ring" class="Ring (strict)"("Visible"=TRUE) -> ()  [unwired: 2 in, 2 out]
                n186 = property on="Test Slider" class="Slide (strict)"("Visible"=FALSE) -> ()  [unwired: 2 in, 2 out]
              }
              frame "Color Enable  **" {
                n187 = Index Array(array=w311, index=4) -> (element=w312:cluster{string[]})
                n188 = call <vilib>:"NT Read String.vi"("Name"=w314) -> ("String"=w313:string)  [unwired: 9 in, 1 out]
                n189 = Unbundle(w312) -> (w308:string[])
                n190 = Match First String(2:w308, 3:w313) -> (0:w309:i32)  [unwired: 1 out]
                n191 = property on="Test Ring" class="Ring (strict)"("Value"=w309, "Strings []"=w308) -> ()  [unwired: 2 in, 2 out]
                n192 = property on="Test Ring" class="Ring (strict)"("Visible"=TRUE) -> ()  [unwired: 2 in, 2 out]
                n193 = property on="Test Slider" class="Slide (strict)"("Visible"=FALSE) -> ()  [unwired: 2 in, 2 out]
              }
              frame Default {
                n194 = property on="Test Ring" class="Ring (strict)"("Visible"=FALSE) -> ()  [unwired: 2 in, 2 out]
                n195 = property on="Test Slider" class="Slide (strict)"("Visible"=FALSE) -> ()  [unwired: 2 in, 2 out]
              }
              frame "Brightness  **", "Color Level  **", "Compression  **", "FPS  **", "Sharpness  **" {
                n196 = call <vilib>:"NT Read Number.vi"("Name"=w320) -> ("Numeric"=w319:dbl)  [unwired: 9 in, 1 out]
                n197 = local write "Test Slider"(w319) -> ()
                n198 = property on="Test Slider" class="Slide (strict)"("Visible"=TRUE, "Scale.Maximum"=100.0 ("Scale.Range:Maximum")) -> ()  [unwired: 2 in, 2 out]
                n199 = property on="Test Ring" class="Ring (strict)"("Visible"=FALSE) -> ()  [unwired: 2 in, 2 out]
              }
            }
          }
        }
        n200 = property on="Progress" class="Clust (strict)"("Visible"=FALSE) -> ()  [unwired: 2 in, 2 out]
      }
      event "Test Name": Mouse Enter {
        # "Populate the ring with the list of tests"
        n201 = event-data() -> ()  [unwired: 1 in, 1 out]
        n202 = call <vilib>:"NT Read String Array.vi"("Name"="/TestMode/TestList") -> ("String Array"=w329:string[])  [unwired: 9 in, 1 out]
        n203 = Build Array (concatenate)("Select the test to run...", w329) -> (w328:string[])
        n204 = property on="Test Name" class="Ring (strict)"("Strings []"=w328) -> ()  [unwired: 2 in, 2 out]
      }
      event "Test Name": Value Change {
        w332 = FALSE ("Visible")
        # "Tell the robot the test name to run"
        n205 = event-data() -> ("NewVal"=w336:u16)  [unwired: 1 in]
        n206 = property on="Test Name" class="Ring (strict)"() -> ("Strings []"=w337:string[])  [unwired: 2 in, 2 out]
        n207 = local write "Progress"(T4 {"Test Progress"=0, "Test Progress Text"=""} ("Progress")) -> ()
        n208 = Index Array(array=w337, index=w336) -> (element=w335:string)
        n209 = call <vilib>:"NT Write String.vi"("String"=w335, "Name"="/TestMode/TestName") -> ()  [unwired: 9 in, 1 out]
        n210 = property on="Progress" class="Clust (strict)"("Visible"=TRUE) -> ()  [unwired: 2 in, 2 out]
        n211 = property on="Motor" class="Clust (strict)"("Visible"=w332) -> ()  [unwired: 2 in, 2 out]
        n212 = property on="Test Slider" class="Slide (strict)"("Visible"=w332) -> ()  [unwired: 2 in, 2 out]
        n213 = property on="On/Off" class="Bool (strict)"("Visible"=w332) -> ()  [unwired: 2 in, 2 out]
        n214 = property on="Rev/Fwd" class="Clust (strict)"("Visible"=w332) -> ()  [unwired: 2 in, 2 out]
        n215 = property on="Test Ring" class="Ring (strict)"("Visible"=w332) -> ()  [unwired: 2 in, 2 out]
      }
      event "Select Auto": Mouse Enter {
        # "Populate the combo box with the list of autonomous options"
        n216 = event-data() -> ()  [unwired: 1 in, 1 out]
        n217 = call <vilib>:"NT Read String Array.vi"("Name"="Auto List") -> ("String Array"=w339:string[])  [unwired: 9 in, 1 out]
        n218 = property on="Select Auto" class="CmbBox"("Strings[]"=w339) -> ()  [unwired: 2 in, 2 out]
      }
      event "Select Auto": Value Change {
        # "User modified the Auto Selection. Write to NT variable so robot knows."
        n219 = event-data() -> ("NewVal"=w343:string)  [unwired: 1 in]
        n220 = call <vilib>:"NT Write String.vi"("String"=w343, "Name"="Auto Selector") -> ()  [unwired: 9 in, 1 out]
      }
      event "Command Selection": Value Change {
        # "Get the params and show in table"
        n221 = event-data() -> ("NewVal"=w350:i32)  [unwired: 1 in]
        n222 = property on="Command Selection" class="MCListbox (strict)"() -> ("ItemNames"=w348:string[][])  [unwired: 2 in, 2 out]
        n223 = call <vilib>:"WPI_DashboardUpdate Command Params.vi"("NewVal"=w350, "Commands"=w348, "Param Tbl"=w349) -> ()  [unwired: 8 in, 1 out]
      }
      event "Execute Command": Value Change {
        # "Started one, Unique ID holds\nresponse"
        n224 = event-data() -> ()  [unwired: 1 in, 1 out]
        n225 = property on="Command Selection" class="MCListbox (strict)"() -> ("ItemNames"=w362:string[][])  [unwired: 2 in, 2 out]
        n226 = Index Array(array=w362, index (row)="Command Selection", index (col)=0) -> (element=w360:string)
        n227 = call <vilib>:"Invoke Commands.vi"("Command Params"="Command Params", "Function Name"=w360) -> ("Params"=w356:u8, "Started"=w355:bool)  [unwired: 7 in, 1 out]
        n228 = Array Subset(array="Command Params", length (row)=w356) -> (w357:string[][])  [unwired: 3 in]
        n229 = Select(t="Executing" ("Cmd Status"), s=w355, f="" ("Cmd Status")) -> (s? t:f=→"Cmd Status":string)
      }
      event "Command Selection": Double Click {
        n230 = event-data() -> ("Row"=w372:i32)  [unwired: 1 in]
        n231 = property on="Command Selection" class="MCListbox (strict)"() -> ("ItemNames"=w375:string[][])  [unwired: 2 in, 2 out]
        n232 = local read "Command Params"() -> (w370:string[][])
        n233 = Index Array(array=w375, index (row)=w372, index (col)=0) -> (element=w373:string)
        n234 = call <vilib>:"Invoke Commands.vi"("Command Params"=w370, "Function Name"=w373) -> ("Params"=w369:u8, "Started"=w364:bool)  [unwired: 7 in, 1 out]
        n235 = Array Subset(array=w370, length (row)=w369) -> (w368:string[][])  [unwired: 3 in]
        n236 = Select(t="Executing" ("Cmd Status"), s=w364, f="" ("Cmd Status")) -> (s? t:f=w365:string)
        n237 = local write "Cmd Status"(w365) -> ()
      }
      event "CheckList": Double Click {
        # "Shift clears all"
        # "Update symbols on the listbox"
        n238 = event-data() -> ("PlatMods.Shift"=w378:bool, "Row"=w380:i32)  [unwired: 1 in]
        n239 = case shown="True" w378 {
          tunnel: w380 -> [w384 _]
          tunnel: 1 -> [w383 _]
          frame False {
            n240 = property on="CheckList" class="LstBox (strict)"() -> ("Item Symbols"=w382:i32[])  [unwired: 2 in, 2 out]
            n241 = Replace Array Subset(array=w382, new element=w383, index=w384) -> (w381:i32[])
            n242 = property on="CheckList" class="LstBox (strict)"("Item Symbols"=w381) -> ()  [unwired: 2 in, 2 out]
          }
          frame True {
            w385 = 0 ("Top Row")
            n243 = property on="CheckList" class="LstBox (strict)"() -> ("Number of Rows"=w387:u32)  [unwired: 2 in, 2 out]
            n244 = Initialize Array(0, w387) -> (w386:i32[])
            n245 = property on="CheckList" class="LstBox (strict)"("Top Row"=w385, "Value"=w385, "Item Symbols"=w386) -> ()  [unwired: 2 in, 2 out]
          }
        }
      }
      event "CheckList": Key Down {
        # "Update symbols on the listbox\nLeft and right keys check and uncheck"
        n246 = event-data() -> ("VKey"=w392:T18)  [unwired: 1 in]
        n247 = case shown="\"Left\", \"Right\"" w392 {
          selector: w392 -> [w397 _]
          tunnel: eventvkey."Left" ("VKey") -> [w395 _]
          frame "Left", "Right" {
            n248 = Equal?(x=w395, y=w397) -> (x = y?=w396:bool)
            n249 = Select(t=0, s=w396, f=1) -> (s? t:f=w398:i32)
            n250 = property on="CheckList" class="LstBox (strict)"() -> ("Item Symbols"=w401:i32[])  [unwired: 2 in, 2 out]
            n251 = Replace Array Subset(array=w401, new element=w398, index="CheckList") -> (w400:i32[])
            n252 = property on="CheckList" class="LstBox (strict)"("Item Symbols"=w400) -> ()  [unwired: 2 in, 2 out]
          }
          frame Default {
          }
        }
      }
      event "DB Camera Config": Value Change {
        # "Show or hide the cluster of controls, store in ini file"
        n253 = event-data() -> ("NewVal"=w406:bool)  [unwired: 1 in]
        n254 = case shown="False" w406 {
          tunnel: w405 -> [w415 _]
          tunnel: [w408 w426] -> w404
          tunnel: w403 -> [w407 w426]
          frame False {
            w422 = "Camera"
            w425 = FALSE ("Visible")
            n255 = local read "Camera Settings"() -> (w414:T2)
            n256 = Index Array(array=w415) -> (element=w418:cluster{string[]})  [unwired: 1 in]
            n257 = Unbundle(w414) -> ("Frame Rate"=w413:i32, "Compression"=w412:i32, "Size"=w416:u16)
            n258 = Unbundle(w418) -> (w417:string[])
            n259 = Index Array(array=w417, index=w416) -> (element=w411:string)
            n260 = call-poly <vilib>:"Write Key.vi"("section"=w422, "value"=w411, "key"="Size", "refnum"=w407) -> ("refnum out"=w424:T16)  [unwired: 2 in, 5 out]
            n261 = call-poly <vilib>:"Write Key.vi"("section"=w422, "value"=w413, "key"="FrameRate", "refnum"=w424) -> ("refnum out"=w423:T16)  [unwired: 1 in, 6 out]
            n262 = property on="Camera Settings" class="Clust (strict)"("Visible"=w425) -> ()  [unwired: 2 in, 2 out]
            n263 = local write "DB Camera Config"(w425) -> ()
            n264 = call-poly <vilib>:"Write Key.vi"("section"=w422, "value"=w412, "key"="Compression", "refnum"=w423) -> ("refnum out"=w409:T16)  [unwired: 1 in, 6 out]
            n265 = call <vilib>:"Close Config Data.vi"("refnum"=w409) -> ("file path"=w410:path)  [unwired: 2 in, 8 out]
            n266 = call <vilib>:"Open Config Data.vi"("configuration file path"=w410) -> ("refnum"=w408:T16)  [unwired: 8 in, 2 out]
          }
          frame True {
            n267 = property on="Camera Settings" class="Clust (strict)"("Visible"=TRUE) -> ()  [unwired: 2 in, 2 out]
          }
        }
      }
      event "Camera Settings": Value Change {
        # "Update summary string when any elements of DB camera change"
        n268 = event-data() -> ("NewVal"=w440:T2)  [unwired: 1 in]
        n269 = Index Array(array=w436) -> (element=w435:cluster{string[]})  [unwired: 1 in]
        n270 = Unbundle(w440) -> ("Frame Rate"=w431:i32, "Compression"=w430:i32, "Size"=w433:u16)
        n271 = Unbundle(w435) -> (w434:string[])
        n272 = Index Array(array=w434, index=w433) -> (element=w432:string)
        n273 = Format Into String(format string="%s   %dfps   %d%%", w432, w431, w430) -> (resulting string=w437:string)  [unwired: 2 in, 1 out]
        n274 = Build Array(w437) -> (w438:string[])
        n275 = property on="DB Camera Config" class="Bool (strict)"("Strings [4]"=w438) -> ()  [unwired: 2 in, 2 out]
      }
      event "Motor.Enable": Value Change {
        # "When the test mode otor enable helper is set, update that\ntree row item's value"
        n276 = event-data() -> ("NewVal"=w447:bool)  [unwired: 1 in]
        n277 = Unbundle("Motor") -> ("Value"=w446:dbl)  [unwired: 1 out]
        n278 = Select(t=w446, s=w447, f=0.0) -> (s? t:f=w444:dbl)
        n279 = call <vilib>:"NT Write Number.vi"("Numeric"=w444, "Name"=w443) -> ()  [unwired: 9 in, 1 out]
      }
      event "Test Slider": Value Change {
        # "When the test mode slider helper is set, update that\ntree row item's value"
        n280 = event-data() -> ("NewVal"=w451:dbl)  [unwired: 1 in]
        n281 = call <vilib>:"NT Write Number.vi"("Numeric"=w451, "Name"=w452) -> ()  [unwired: 9 in, 1 out]
      }
      event "On/Off": Value Change {
        # "When the test mode on/off helper value is set, update that\ntree row item's value"
        n282 = event-data() -> ("NewVal"=w457:bool)  [unwired: 1 in]
        n283 = Boolean To (0,1)(Boolean=w457) -> (0, 1=w456:i16)
        n284 = call <vilib>:"NT Write Number.vi"("Numeric"=w456, "Name"=w455) -> ()  [unwired: 9 in, 1 out]
      }
      event "Rev/Fwd": Value Change {
        # "When the test mode helper value for relays is set, update that\ntree row item's value"
        n285 = event-data() -> ("NewVal.Forward"=w466:bool, "NewVal.Reverse"=w465:bool)  [unwired: 1 in]
        n286 = Boolean To (0,1)(Boolean=w466) -> (0, 1=w462:i16)
        n287 = Boolean To (0,1)(Boolean=w465) -> (0, 1=w464:i16)
        n288 = Negate(x=w464) -> (-x=w463:i16)
        n289 = Add(x=w462, y=w463) -> (x+y=w461:i16)
        n290 = call <vilib>:"NT Write Number.vi"("Numeric"=w461, "Name"=w460) -> ()  [unwired: 9 in, 1 out]
      }
      event "Test Ring": Value Change {
        # "When a test mode helper value is selected from the ring,\nset the tree item's variable to the string value"
        n291 = event-data() -> ("NewVal"=w471:u16)  [unwired: 1 in]
        n292 = property on="Test Ring" class="Ring (strict)"() -> ("Strings []"=w472:string[])  [unwired: 2 in, 2 out]
        n293 = Index Array(array=w472, index=w471) -> (element=w470:string)
        n294 = call <vilib>:"NT Write String.vi"("String"=w470, "Name"=w469) -> ()  [unwired: 9 in, 1 out]
      }
      event "Rec Mode": Value Change {
        # "Update globals for recording mode and path to read log from.\nClear when logging and let NetworkTables set path for vision to\nuse."
        n295 = event-data() -> ("NewVal"=w484:enum32{"Stop", "Record", "Playback"})  [unwired: 1 in]
        n296 = global write "WPI_DashboardLogging Global.vi" "Logging Filename"(path "") -> ()
        n297 = global write "WPI_DashboardLogging Global.vi" "Recording"(w484) -> ()
        n298 = case shown="\"Playback\"" w484 {
          tunnel: w483 -> [_ w486 w495]
          tunnel: [_ _ w494] -> w480
          tunnel: [_ _ w493] -> _
          tunnel: w478 -> [_ _ w491]
          tunnel: cluster{i32, i32} {-250, 170} -> [_ _ w490]
          tunnel: [_ _ T19 {"Image Size"=TRUE, "Image Type"=TRUE, "Pixel Value"=TRUE, "ROI Information"=TRUE, "Zoom Factor"=FALSE} ("Image Information Shown:All Elements")] -> w476
          tunnel: [_ _ TRUE ("Zoom Factor")] -> w475
          tunnel: w474 -> [_ _ w487]
          frame Default {
          }
          frame "Stop", "Record" {
            # "Place Window too"
            n299 = invoke class="VI" method="FP.Close"(reference=w486) -> (reference out=w485:refnum<vi>)  [unwired: 2 in, 2 out]
            n300 = invoke class="VI" method="Abort VI"(reference=w485) -> ()  [unwired: 2 in, 3 out]
          }
          frame "Playback" {
            n301 = call "Open Playback Panel.vi"("Offset"=w490, "DB VI Ref"=w491, "Playback in"=w495) -> ("Playback out"=w492:refnum<vi>)  [unwired: 8 in]
            n302 = register-events(w492, w487) -> (reference out=w494:refnum<event-registration>, error out=w493:errorcluster)  [unwired: 2 in]
          }
        }
        n303 = property on="Camera Image" class="ImageControl"("Image Information Shown"=w476, "Image Information Visible"=w475) -> ()  [unwired: 2 in, 2 out]
        n304 = call <vilib>:"WPI_DashboardNT Log FieldName Cache.vi"("Operation"=enum16{"Lookup/Add", "Index", "Clear"}."Clear") -> ()  [unwired: 8 in, 3 out]
      }
      event Panel Close {
        w497 = enum32{"Stop", "Record", "Playback"}."Stop" ("Rec Mode")
        # "Playback window has been closed, abort"
        n305 = event-data() -> ()  [unwired: 1 in, 4 out]
        n306 = local write "Rec Mode"(w497) -> ()
        n307 = global write "WPI_DashboardLogging Global.vi" "Recording"(w497) -> ()
      }
      event Panel Close {
        # "Abort playback window and ourself"
        n308 = event-data() -> ()  [unwired: 1 in, 4 out]
        n309 = invoke class="VI" method="FP.Close"(reference=w503) -> (reference out=w502:refnum<vi>)  [unwired: 2 in, 2 out]
        n310 = invoke class="VI" method="Abort VI"(reference=w502) -> (error out=w501:errorcluster)  [unwired: 2 in, 2 out]
        n311 = invoke class="VI" method="Abort VI"(error in=w501) -> ()  [unwired: 2 in, 3 out]
      }
      event User Event {
        n312 = event-data() -> ("IDs"=w511:cluster{"RPC field ID":u16, "Unique ID":u16}, "String"=w510:string)  [unwired: 1 in]
        n313 = Bundle("IDs"=w511, "String"=w510) -> (w509:T6)  [unwired: 1 in]
        n314 = call <vilib>:"Retrieve RPC Response.vi"("RPC Response"=w509) -> ("Output"=w506:string[][])  [unwired: 10 in]
        n315 = Build Array (concatenate)(w504, w506) -> (w505:string[][])
        n316 = local write "Command Params"(w505) -> ()
        n317 = local write "Cmd Status"("" ("Cmd Status")) -> ()
      }
      event "Vision": Value Change {
        # "Enable/Disable Compression slider.\nHW USB is hard-coded into the camera"
        n318 = event-data() -> ("NewVal"=w518:u16)  [unwired: 1 in]
        n319 = Equal?(x=w518, y=u32 2 ("milliseconds to wait")) -> (x = y?=w516:bool)
        n320 = Select(t=T20."Disabled and Grayed Out" ("Disabled"), s=w516, f=T20."Enabled" ("Disabled")) -> (s? t:f=w513:T20)
        n321 = property on="Compression" class="Slide (strict)"("DisabledEnum"=w513) -> ()  [unwired: 2 in, 2 out]
      }
      event "Tree": Double Click {
        n322 = event-data() -> ("PlatMods"=w523:T23, "Tag"=w522:string)  [unwired: 1 in]
        n323 = Unbundle(w523) -> ("Shift"=w521:bool)  [unwired: 4 out]
        n324 = Not(x=w521) -> (.not. x?=w520:bool)
        n325 = call <vilib>:"NT Update Persistence.vi"("Persistence"=w520, "Name"=w522) -> ()  [unwired: 9 in, 1 out]
      }
    }
  }
  n326 = while {
    tunnel: w51 -> [w527]
    i -> [w530]
    stop <- FALSE stop-if-true
    n327 = Wait (ms)(milliseconds to wait=u32 100) -> ()  [unwired: 1 out]
    n328 = case shown="\"Playback\"" "Rec Mode" {
      tunnel: w530 -> [_ _ w545]
      tunnel: [u32 2829099 ("Base Color") u32 11141120 ("Target Color") w534] -> w526
      frame "Stop", Default {
        # "Reset the color, extra updates don't cost much"
      }
      frame "Record" {
      }
      frame "Playback" {
        # "Playback"
        n329 = Quotient & Remainder(x=w545, y=u32 50 ("milliseconds to wait")) -> (x-y*floor(x/y)=w541:u32)  [unwired: 1 out]
        n330 = Divide(x=w541, y=u32 50 ("milliseconds to wait")) -> (x/y=w538:dbl)
        n331 = Multiply(x=6.283185307179586, y=w538) -> (x*y=w543:dbl)
        n332 = Sine(x=w543) -> (sin(x)=w542:dbl)
        n333 = Absolute Value(x=w542) -> (abs(x)=w535:dbl)
        n334 = call "Interpolate RGB Color.vi"("Proportion"=w535, "Target Color"=u32 30976, "Base Color"=u32 2829099) -> ("Result Color"=w534:u32)  [unwired: 8 in]
      }
    }
    n335 = property class="Pane"(reference=w527, "PaneColor"=w526) -> ()  [unwired: 1 in, 2 out]
  }
  n336 = local write "Dashboard Tab"(T1."Drive" ("Dashboard Tab")) -> ()
  n337 = property on="On/Off" class="Bool (strict)"("Visible"=w19) -> ()  [unwired: 2 in, 2 out]
  n338 = property on="Motor" class="Clust (strict)"("Visible"=w19) -> ()  [unwired: 2 in, 2 out]
  n339 = property on="Progress" class="Clust (strict)"("Visible"=w19) -> ()  [unwired: 2 in, 2 out]
  n340 = property on="Test Ring" class="Ring (strict)"("Visible"=w19) -> ()  [unwired: 2 in, 2 out]
  n341 = property on="Rev/Fwd" class="Clust (strict)"("Visible"=w19) -> ()  [unwired: 2 in, 2 out]
  n342 = property on="Camera Settings" class="Clust (strict)"("Visible"=w19) -> ()  [unwired: 2 in, 2 out]
  n343 = while {
    tunnel: u16 1741 ("timeout ms (25000)") -> [w547]
    stop <- FALSE stop-if-true
    n344 = TCP Create Listener(10:w547) -> (0:w546:errorcluster, 3:w548:refnum<k5>)  [unwired: 4 in, 1 out]
    n345 = case shown="No Error" w546 {
      selector: w546 -> [w550 _]
      tunnel: w548 -> [w551 _]
      frame No Error {
        n346 = while {
          tunnel: w551 -> [w554]
          tunnel: w550 -> [w553]
          stop <- FALSE stop-if-true
          n347 = TCP Wait On Listener(8:w553, 11:w554) -> (0:w555:errorcluster, 4:w556:refnum<k5>)  [unwired: 2 in, 3 out]
          n348 = local write "TCP"(w556) -> ()
          n349 = case shown="No Error" w555 {
            frame No Error {
            }
            frame Error {
              n350 = Wait (ms)(milliseconds to wait=u32 1000) -> ()  [unwired: 1 out]
            }
          }
        }
      }
      frame Error {
        n351 = Wait (ms)(milliseconds to wait=u32 1000) -> ()  [unwired: 1 out]
      }
    }
  }
  n352 = local write "DB Camera Config"(w19) -> ()
  n353 = local write "Command Params"(string[][] [] ("Command Params")) -> ()
  n354 = global write "WPI_DashboardLogging Global.vi" "Recording"(w45) -> ()
  n355 = local write "Command Selection"(u16 0 ("milliseconds to wait")) -> ()
  n356 = local write "Rec Mode"(w45) -> ()
